vi "Calculate Background IA.vi"(4 "Fit Params":cluster{"slope":sgl, "zero":sgl}={"slope"=1.0, "zero"=0.0}, 6 "Sw From Spk":bool, 8 "error in":errorcluster, 9 "Wait":i32=5, 10 "Filter":bool, 11 "Cell Data in":refnum<class "PAS Cell Data.lvclass">) -> (0 "error out":errorcluster, 3 "Cell Data out":refnum<class "PAS Cell Data.lvclass">)   [LabVIEW 2016, in "PAS Library.lvlib" / "PAS Cell Data.lvclass"]
doc: "Calculate a running average of the IA when the filter is ON. The running average is pumped into the member <b>IABackground</b>. The first time after a filter switch, there is nothing to average - the background will just be the current value. After this, the background is calculated in a running average as this:\n\nIABackground = (IABackground(avg)*Number_Averaged + IA)/(Number_Averaged+1)\n\nThis will provide a current background of IA for calculating a background corrected absorption over the next sample period."
uses:
  PAS Cell Data.lvclass
  PAS Cell Data.lvclass/PAS Cell Data.ctl
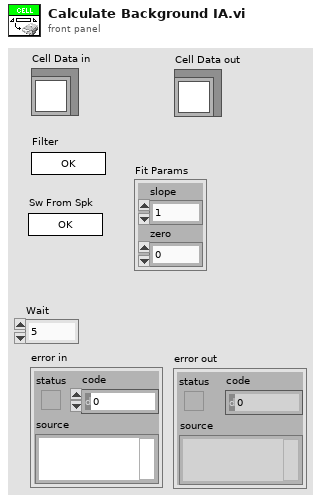
[diagram p1: front panel]
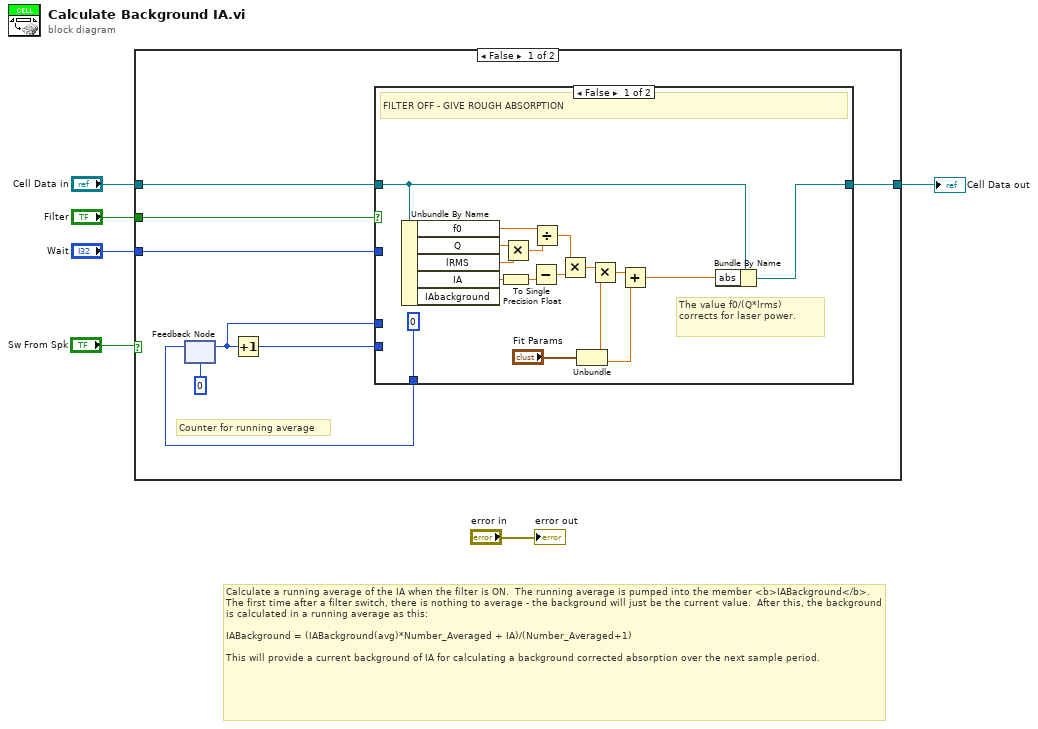
[diagram p0: block diagram]
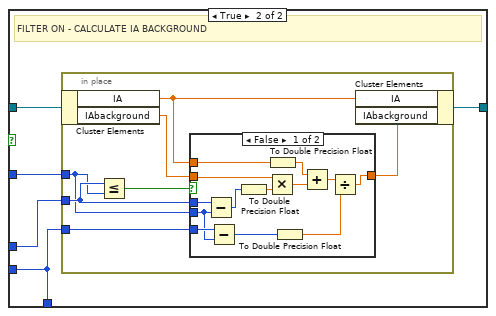
[diagram p2: hidden frame]
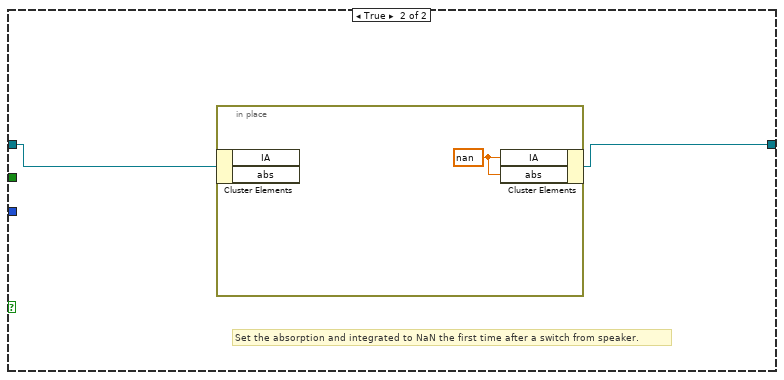
[diagram p4: hidden frame]
diagram:
  # "Calculate a running average of the IA when the filter is ON.  The running average is pumped into the member <b>IABackground</b>.  The first time after a filter switch, there is nothing to average - the background will just be the current value.  After this, the background is calculated in a running average as this:\n\nIABackground = (IABackground(avg)*Number_Averaged + IA)/(Number_Averaged+1)\n\nThis will provide a current background of IA for calculating a background corrected absorption over the next sample period."
  n1 = case shown="False" "Sw From Spk" {
    tunnel: "Cell Data in" -> [w13 w60]
    tunnel: "Filter" -> [w12 _]
    tunnel: "Wait" -> [w8 _]
    tunnel: [w7 w59] -> w2
    frame False {
      # "Counter for running average"
      n2 = feedback #1(0) -> (w10:i32)
      n3 = Increment(x=w10) -> (x+1=w11:i32)
      n4 = case shown="False" w12 {
        tunnel: w13 -> [w31 w37]
        tunnel: w11 -> [_ w34]
        tunnel: w10 -> [_ w36]
        tunnel: [0 w34] -> w9
        tunnel: [w30 w35] -> w7
        tunnel: w8 -> [_ w33]
        frame False {
          # "The value f0/(Q*lrms) corrects for laser power."
          # "FILTER OFF - GIVE ROUGH ABSORPTION"
          n5 = Unbundle By Name(w31) -> ("f0"=w29:sgl, "Q"=w17:sgl, "lRMS"=w16:dbl, "IA"=w28:sgl, "IAbackground"=w23:dbl)
          n6 = To Single Precision Float(number=w23) -> (single precision float=w24:sgl)
          n7 = Multiply(x=w17, y=w16) -> (x*y=w15:dbl)
          n8 = Subtract(x=w28, y=w24) -> (x-y=w27:sgl)
          n9 = Divide(x=w29, y=w15) -> (x/y=w26:dbl)
          n10 = Multiply(x=w26, y=w27) -> (x*y=w25:dbl)
          n11 = Unbundle("Fit Params") -> ("slope"=w19:sgl, "zero"=w18:sgl)
          n12 = Multiply(x=w25, y=w19) -> (x*y=w22:dbl)
          n13 = Add(x=w22, y=w18) -> (x+y=w21:dbl)
          n14 = Bundle By Name(cluster=w31, "abs"=w21) -> (w30:refnum<class "PAS Cell Data.lvclass">)
        }
        frame True {
          # "FILTER ON - CALCULATE IA BACKGROUND"
          n15 = in-place {
            in-place-border: w36 -> [w40]
            in-place-border: w34 -> [w41]
            in-place-border: w33 -> [w38]
            n16 = in-place-cluster #2(w37) -> ("IA"=w44:sgl, "IAbackground"=w43:dbl)
            n17 = Less Or Equal?(x=w40, y=w38) -> (x <= y?=w39:bool)
            n18 = case shown="False" w39 {
              tunnel: w43 -> [w57 w58]
              tunnel: w44 -> [w50 _]
              tunnel: [w54 w58] -> w42
              tunnel: w40 -> [w49 _]
              tunnel: w41 -> [w47 _]
              tunnel: w38 -> [w46 _]
              frame False {
                n19 = Subtract(x=w49, y=w46) -> (x-y=w48:i32)
                n20 = Subtract(x=w47, y=w46) -> (x-y=w45:i32)
                n21 = To Double Precision Float(number=w48) -> (double precision float=w53:dbl)
                n22 = Multiply(x=w57, y=w53) -> (x*y=w56:dbl)
                n23 = To Double Precision Float(number=w50) -> (double precision float=w51:dbl)
                n24 = To Double Precision Float(number=w45) -> (double precision float=w52:dbl)
                n25 = Add(x=w51, y=w56) -> (x+y=w55:dbl)
                n26 = Divide(x=w55, y=w52) -> (x/y=w54:dbl)
              }
              frame True {
              }
            }
            n27 = in-place-cluster #2("IA"=w44, "IAbackground"=w42) -> (w35:refnum<class "PAS Cell Data.lvclass">)
          }
        }
      }
      n28 = feedback-in #1(w9) -> ()
    }
    frame True {
      # "Set the absorption and integrated to NaN the first time after a switch from speaker."
      n29 = in-place {
        w61 = sgl nan ("derived.IA")
        n30 = in-place-cluster #3(w60) -> ()  [unwired: 2 out]
        n31 = in-place-cluster #3("IA"=w61, "abs"=w61) -> (w59:refnum<class "PAS Cell Data.lvclass">)
      }
    }
  }
  "Cell Data out" <- w2
  "error out" <- "error in"
